vi "OUTPUT2sql.vi"() -> ()   [LabVIEW 2015]
uses:
  Controls/STORE_INPUT_NO_CLUSTER.ctl
  Controls/STORE_INPUT_INFORMATION_Cluster.ctl
  <vilib>/addons/database/Connection.llb/DB Tools Open Connec (String).vi
  <vilib>/addons/database/Connection.llb/Conn Execute.vi
  <vilib>/addons/database/Recordset.llb/Rec Destroy - Connection.vi
  <vilib>/addons/database/_DB Variant To Data/Database Variant To Data.xnode
  <vilib>/addons/database/NI_Database_API.lvlib
panel:
  out "Numeric 2":i32
  in  "stop":bool
  out "error out 5":errorcluster
  out "Numeric":i32
  out "error out 4":errorcluster
  out "error out 3":errorcluster
  out "error out 2":errorcluster
  out "error out":errorcluster
  out "Find Array":i32[](array[numeric])
  out "Input No.":string
  out "Table 2":string[][](table)
  out "ECODE":string
  in  "Input Date":timestamp format="%<%d/%m/%Y>T"
  in  "Browse":path=path "\\\\192.168.1.45\\Du Lieu Kho/Data/OutLine" caption="Path"
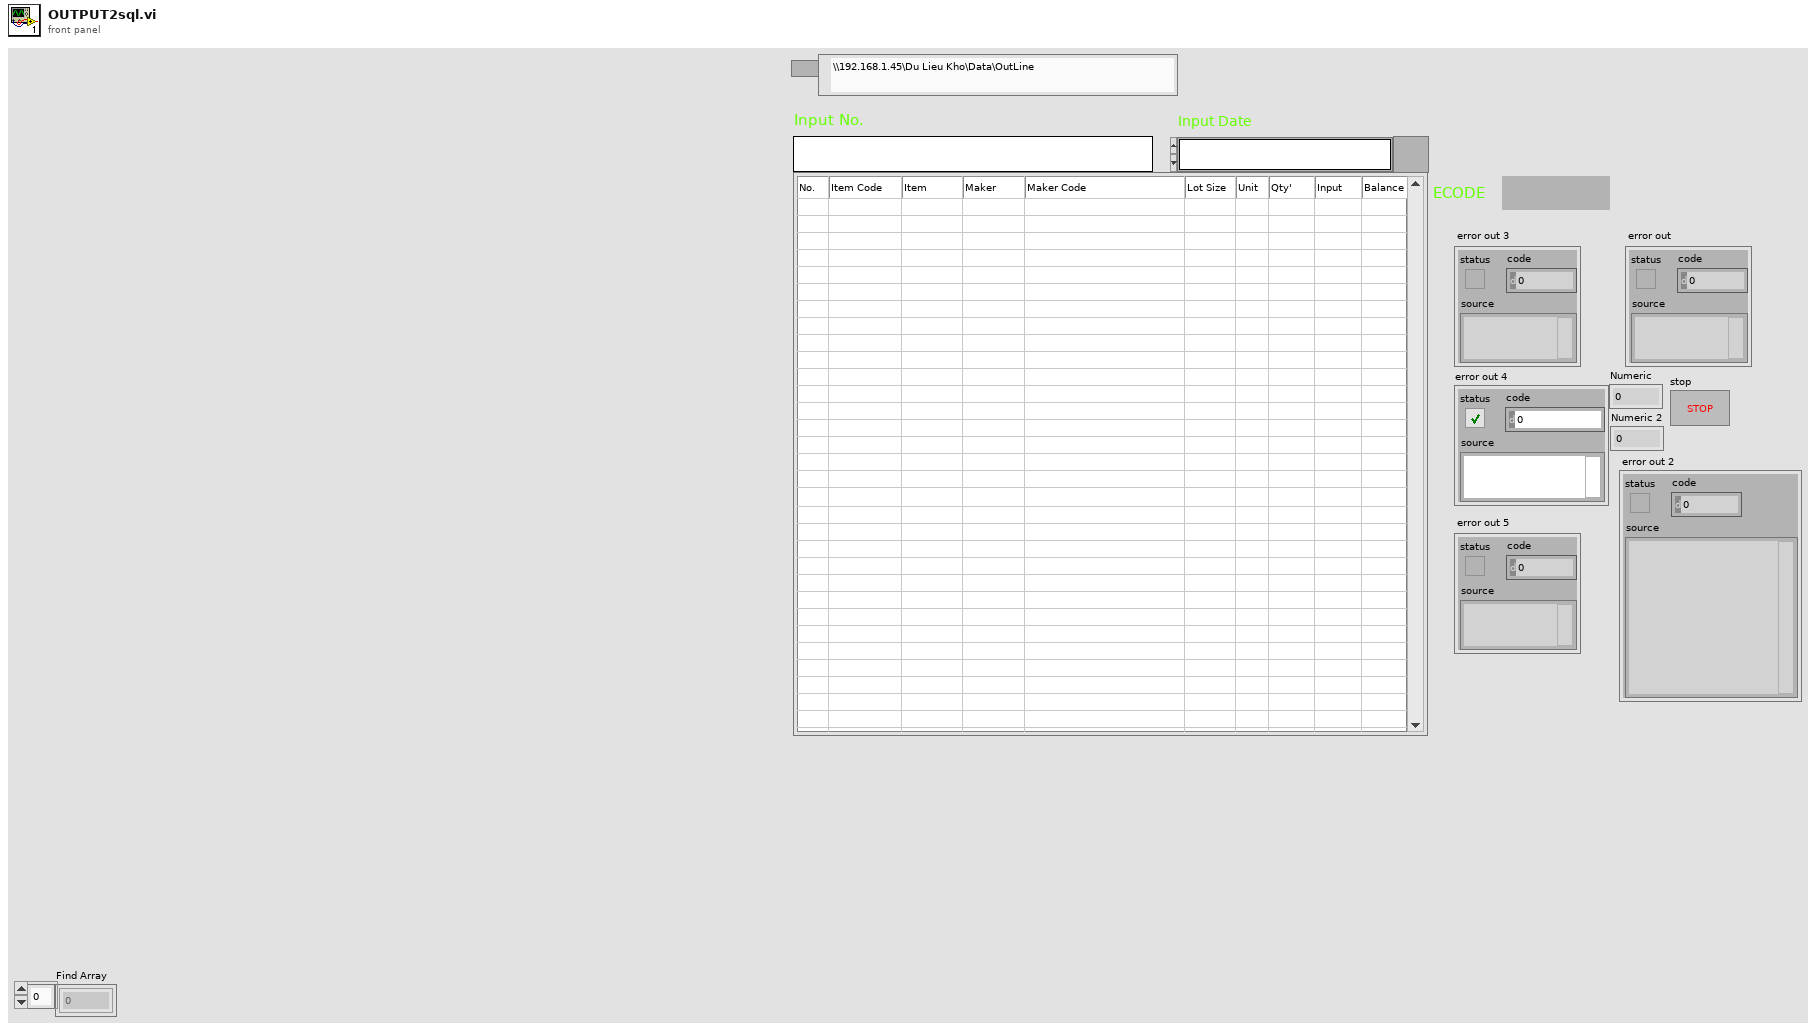
[diagram p1: front panel]
types:
  T1 = typedef "STORE_INPUT_NO_CLUSTER.ctl" = cluster{"NO":dbl, "ITEM_CODE":string, "ITEM":string, "MAKER":string, "MAKER_CODE":string, "LOT_SIZE":dbl, "UNIT":string, "QUANTITY":dbl, "INPUT":dbl, "BALANCE":dbl, "DESTINATION":string, "INVOICE_NO":string}
  T2 = enum16{"open", "replace", "create", "open or create", "replace or create", "replace or create with confirmation"}
  T3 = typedef "STORE_INPUT_INFORMATION_Cluster.ctl" = cluster{"INPUT_NO":string, "INPUT_DATE":timestamp, "ECODE":string}
  T4 = typedef "NI_Database_API.lvlib/Conn ObjectReference.ctl" = refnum<k1>
  T5 = typedef "NI_Database_API.lvlib/Rec ObjectReference.ctl" = refnum<k1>
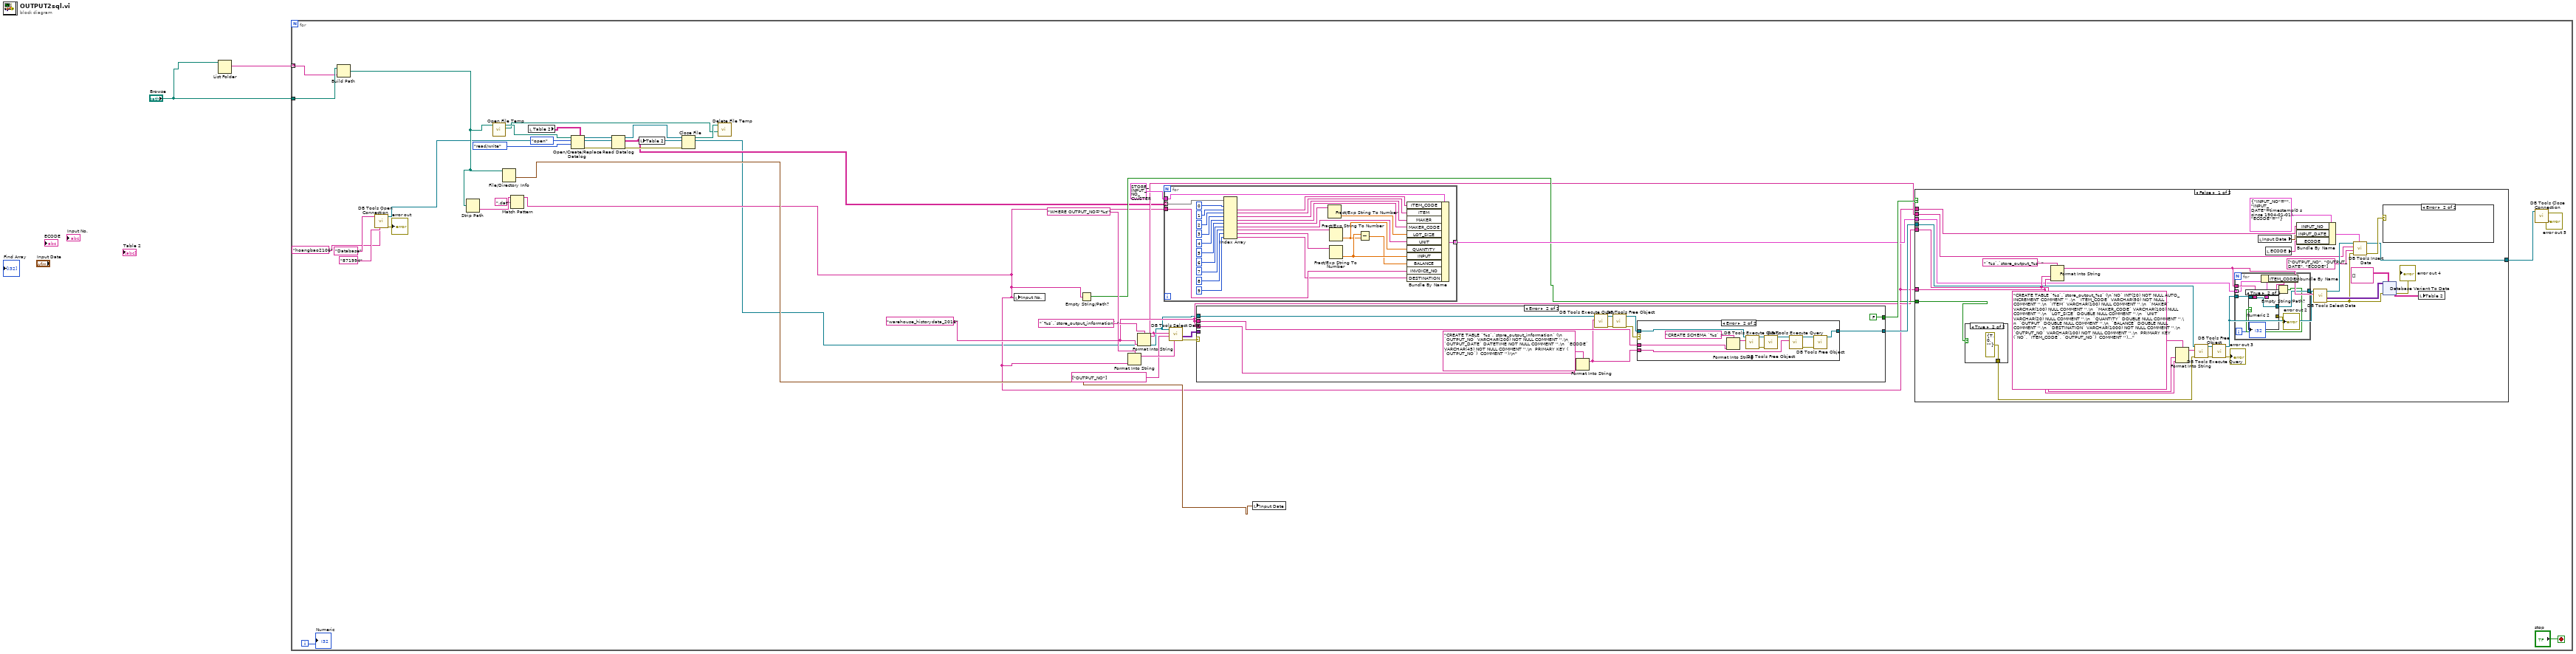
[diagram p0: block diagram]
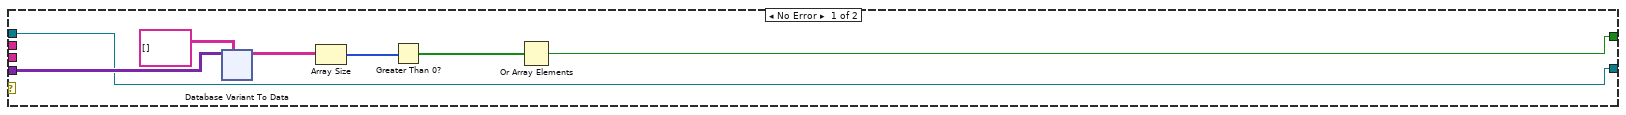
[diagram p2: hidden frame]
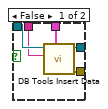
[diagram p6: hidden frame]
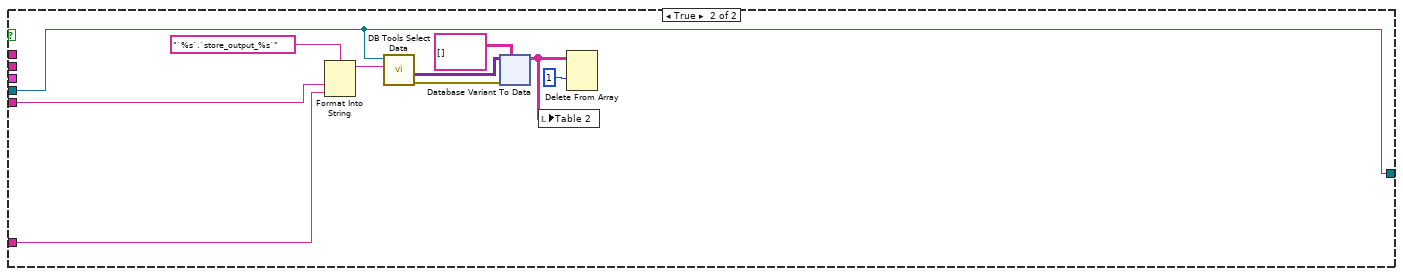
[diagram p7: hidden frame]
diagram:
  n1 = List Folder(path="Browse") -> (filenames=w2:string[])  [unwired: 3 in, 3 out]
  n2 = for {
    tunnel: "Browse" -> [w14]
    tunnel: w2 -> [w13] mode=indexing
    i -> [w11]
    stop <- "stop" stop-if-true
    w21 = "warehouse_historydata_2016"
    n3 = Build Path(base path=w14, name or relative path=w13) -> (appended path=w12:path)
    n4 = call-poly <vilib>:"DB Tools Open Connection.vi"("password"="871994" ("userID"), "userID"="hoangbao2106", "connection information"="Database" ("userID")) -> ("error out"=→"error out":errorcluster, "connection reference"=w6:T4)  [unwired: 5 in]
    n5 = Strip Path(path=w12) -> (name=w18:string)  [unwired: 1 out]
    n6 = call "Open File Temp.vi"("Path file"=w12) -> ("Source Path"=w33:path, "Temp path"=w35:path)  [unwired: 7 in, 2 out]
    n7 = File/Directory Info(path=w12) -> (last mod=w19:timestamp)  [unwired: 1 in, 6 out]
    n8 = Match Pattern(string=w18, regular expression=".dat") -> (before substring=w15:string)  [unwired: 1 in, 3 out]
    n9 = local read "Table 2"() -> (w42:string[][])
    n10 = Open/Create/Replace Datalog(5:w42, 9:enum16{"read/write", "read-only", "write-only"}."read/write" ("access (0:read/write)"), 10:T2."open" ("operation (0:open)"), 11:w35) -> (0:w37:errorcluster, 3:w39:refnum<k1>)  [unwired: 2 in, 1 out]
    n11 = Read Datalog(4:w37, 7:w39) -> (0:w36:errorcluster, 2:w16:string[][], 3:w38:refnum<k1>)  [unwired: 1 in]
    n12 = local write "Table 2"(w16) -> ()
    n13 = Close File(refnum=w38, error in=w36) -> (path=w34:path)  [unwired: 1 out]
    n14 = call "Delete File Temp.vi"("Source Path"=w33, "Temp path"=w34) -> ()  [unwired: 8 in, 2 out]
    n15 = local write "Input No."(w15) -> ()
    n16 = Empty String/Path?(string/path=w15) -> (empty?=w23:bool)
    n17 = Format Into String(format string="WHERE OUTPUT_NO='%s'", w15) -> (resulting string=w31:string)  [unwired: 2 in, 1 out]
    n18 = Format Into String(format string="`%s`.`store_output_information` ", w21) -> (resulting string=w20:string)  [unwired: 2 in, 1 out]
    n19 = for {
      tunnel: w16 -> [w68] mode=indexing
      tunnel: T1 {"NO"=0.0, "ITEM_CODE"="", "ITEM"="", "MAKER"="", "MAKER_CODE"="", "LOT_SIZE"=0.0, "UNIT"="", "QUANTITY"=0.0, "INPUT"=0.0, "BALANCE"=0.0, "DESTINATION"="", "INVOICE_NO"=""} -> [w69]
      tunnel: [w48] -> w24 mode=indexing
      tunnel: w15 -> [w47]
      n20 = Index Array(array=w68, index #1=0 ("index"), index #2=1 ("index"), index #3=2 ("index"), index #4=3 ("index"), index #5=4 ("index"), index #6=5 ("index"), index #7=6 ("index"), index #8=7 ("index"), index #9=8 ("index"), index #10=9 ("index")) -> (element #2=w57:string, element #3=w56:string, element #4=w55:string, element #5=w54:string, element #6=w53:string, element #7=w51:string, element #8=w50:string, element #9=w49:string, element #10=w43:string)  [unwired: 1 out]
      n21 = Fract/Exp String To Number(string=w53) -> (number=w52:dbl)  [unwired: 3 in, 1 out]
      n22 = Fract/Exp String To Number(string=w50) -> (number=w45:dbl)  [unwired: 3 in, 1 out]
      n23 = Fract/Exp String To Number(string=w49) -> (number=w46:dbl)  [unwired: 3 in, 1 out]
      n24 = Subtract(x=w46, y=w45) -> (x-y=w44:dbl)
      n25 = Bundle By Name(cluster=w69, "ITEM_CODE"=w57, "ITEM"=w56, "MAKER"=w55, "MAKER_CODE"=w54, "LOT_SIZE"=w52, "UNIT"=w51, "QUANTITY"=w45, "INPUT"=w46, "BALANCE"=w44, "INVOICE_NO"=w47, "DESTINATION"=w43) -> (w48:T1)
    }
    n26 = call <vilib>:"DB Tools Select Data.vi"("condition"=w31, "columns"=string[] ["OUTPUT_NO"], "table"=w20, "connection reference"=w6) -> ("error out"=w27:errorcluster, "data"=w30:variant[][])  [unwired: 2 in, 1 out]
    n27 = case shown="Error" w27 {
      tunnel: w30 -> [w76 _]
      tunnel: [w71 FALSE] -> w28
      tunnel: w6 -> [w70 w128]
      tunnel: [w70 w124] -> w26
      tunnel: w21 -> [_ w126]
      tunnel: w21 -> [_ w122]
      frame No Error {
        n28 = xnode "Database Variant To Data"("database variant"=w76, "type"=string[][] []) -> ("data"=w74:string[][])  [unwired: 1 in, 1 out]
        n29 = Array Size(array=w74) -> (size(s)=w73:i32[])
        n30 = Greater Than 0?(x=w73) -> (x > 0?=w72:bool[])
        n31 = Or Array Elements(Boolean array=w72) -> (logical OR=w71:bool)
      }
      frame Error {
        n32 = Format Into String(format string="CREATE TABLE `%s`.`store_output_information` (\n  `OUTPUT_NO` VARCHAR(200) NOT NULL COMMENT '',\n  `OUTPUT_DATE` DATETIME NOT NULL COMMENT '',\n  `ECODE` VARCHAR(45) NOT NULL COMMENT '',\n  PRIMARY KEY (  `OUTPUT_NO`)  COMMENT '');\n", w122) -> (resulting string=w121:string)  [unwired: 2 in, 1 out]
        n33 = call-poly <vilib>:"DB Tools Execute Query.vi"("SQL query"=w121, "connection reference"=w128) -> ("error out"=w130:errorcluster, "recordset reference"=w131:T5)  [unwired: 6 in]
        n34 = call-poly <vilib>:"DB Tools Free Object.vi"("error in (no error)"=w130, "recordset reference"=w131) -> ("error out"=w127:errorcluster, "connection reference"=w125:T4)  [unwired: 8 in]
        n35 = case shown="Error" w127 {
          tunnel: w125 -> [w132 w143]
          tunnel: w126 -> [_ w141]
          tunnel: w121 -> [_ w135]
          tunnel: [w132 w134] -> w124
          frame No Error {
          }
          frame Error {
            n36 = Format Into String(format string="CREATE SCHEMA `%s` ;" ("SQL query"), w141) -> (resulting string=w133:string)  [unwired: 2 in, 1 out]
            n37 = call-poly <vilib>:"DB Tools Execute Query.vi"("SQL query"=w133, "connection reference"=w143) -> ("error out"=w139:errorcluster, "recordset reference"=w140:T5)  [unwired: 6 in]
            n38 = call-poly <vilib>:"DB Tools Free Object.vi"("error in (no error)"=w139, "recordset reference"=w140) -> ("connection reference"=w136:T4)  [unwired: 8 in, 1 out]
            n39 = call-poly <vilib>:"DB Tools Execute Query.vi"("SQL query"=w135, "connection reference"=w136) -> ("error out"=w138:errorcluster, "recordset reference"=w137:T5)  [unwired: 6 in]
            n40 = call-poly <vilib>:"DB Tools Free Object.vi"("error in (no error)"=w138, "recordset reference"=w137) -> ("connection reference"=w134:T4)  [unwired: 8 in, 1 out]
          }
        }
      }
    }
    n41 = local write "Input Date"(w19) -> ()
    n42 = case shown="False" w28 {
      tunnel: w26 -> [w172 w241]
      tunnel: w21 -> [w167 w235]
      tunnel: w15 -> [w166 w236]
      tunnel: [w155 w241] -> w5
      tunnel: w24 -> [w165 _]
      tunnel: w20 -> [w158 _]
      tunnel: w15 -> [w154 _]
      tunnel: w23 -> [w148 _]
      frame False {
        n43 = case shown="True" w148 {
          tunnel: [_ errorcluster {"status"=TRUE, "code"=0, "source"=""} ("error constant")] -> w147
          frame False {
          }
          frame True {
          }
        }
        n44 = Format Into String(format string="`%s`.`store_output_%s` " ("SQL query"), w167, w166) -> (resulting string=w161:string)  [unwired: 2 in, 1 out]
        n45 = Format Into String(format string="CREATE TABLE `%s`.`store_output_%s` (\n`NO` INT(20) NOT NULL AUTO_INCREMENT COMMENT '' ,\n  `ITEM_CODE` VARCHAR(50) NOT NULL COMMENT '',\n  `ITEM` VARCHAR(100) NULL COMMENT '',\n  `MAKER` VARCHAR(100) NULL COMMENT '',\n  `MAKER_CODE` VARCHAR(100) NULL COMMENT '',\n  `LOT_SIZE` DOUBLE NULL COMMENT '',\n  `UNIT` VARCHAR(20) NULL COMMENT '',\n  `QUANTITY` DOUBLE NULL COMMENT '',\n  `OUTPUT` DOUBLE NULL COMMENT '',\n  `BALANCE` DOUBLE NULL COMMENT '',\n  `DESTINATION` VARCHAR(1000) NOT NULL COMMENT '',\n  `OUTPUT_NO` VARCHAR(100) NOT NULL COMMENT '',\n  PRIMARY KEY (`NO`, `ITEM_CODE`, `OUTPUT_NO`)  COMMENT '');\n" ("SQL query"), w167, w166) -> (resulting string=w160:string)  [unwired: 2 in, 1 out]
        n46 = call-poly <vilib>:"DB Tools Execute Query.vi"("error in (no error)"=w147, "SQL query"=w160, "connection reference"=w172) -> ("error out"=w169:errorcluster, "recordset reference"=w170:T5)  [unwired: 5 in]
        n47 = call-poly <vilib>:"DB Tools Free Object.vi"("error in (no error)"=w169, "recordset reference"=w170) -> ("error out"=→"error out 3":errorcluster, "connection reference"=w146:T4)  [unwired: 8 in]
        n48 = for {
          tunnel: w146 -> [w225]
          tunnel: w161 -> [w224]
          tunnel: w165 -> [w221] mode=indexing
          tunnel: [w223] -> _
          i -> [w218]
          n49 = Unbundle By Name(w221) -> ("ITEM_CODE"=w220:string)
          n50 = Empty String/Path?(string/path=w220) -> (empty?=w219:bool)
          n51 = case shown="True" w219 {
            tunnel: w225 -> [w230 w231]
            tunnel: w224 -> [w229 _]
            tunnel: [w228 w231] -> w223
            tunnel: [w227 _] -> w222
            tunnel: w221 -> [w226 _]
            frame False {
              n52 = call <vilib>:"DB Tools Insert Data.vi"("data"=w226, "table"=w229, "connection reference"=w230) -> ("error out"=w227:errorcluster, "connection reference out"=w228:T4)  [unwired: 7 in]
            }
            frame True {
            }
          }
          "error out 2" <- w222
          "Numeric 2" <- w218
        }
        n53 = local read "Input Date"() -> (w153:timestamp)
        n54 = local read "ECODE"() -> (w152:string)
        n55 = Bundle By Name(cluster=T3 {"INPUT_NO"="", "INPUT_DATE"=timestamp(0 s since 1904-01-01), "ECODE"=""} ("INVOICE_INFORMATION_Cluster"), "INPUT_NO"=w154, "INPUT_DATE"=w153, "ECODE"=w152) -> (w151:T3)
        n56 = call <vilib>:"DB Tools Select Data.vi"("table"=w161, "connection reference"=w146) -> ("error out"=w157:errorcluster, "data"=w164:variant[][], "connection reference out"=w159:T4)  [unwired: 4 in]
        n57 = call <vilib>:"DB Tools Insert Data.vi"("data"=w151, "error in (no error)"=w157, "columns"=string[] ["OUTPUT_NO", "OUTPUT_DATE", "ECODE"], "table"=w158, "connection reference"=w159) -> ("error out"=w156:errorcluster, "connection reference out"=w155:T4)  [unwired: 5 in]
        n58 = case shown="Error" w156 {
          frame No Error {
          }
          frame Error {
          }
        }
        n59 = xnode "Database Variant To Data"("database variant"=w164, "error in (no error)"=w157, "type"=string[][] []) -> ("data"=w162:string[][], "error out"=→"error out 4":errorcluster)
        n60 = local write "Table 2"(w162) -> ()
      }
      frame True {
        n61 = Format Into String(format string="`%s`.`store_output_%s`", w235, w236) -> (resulting string=w234:string)  [unwired: 2 in, 1 out]
        n62 = call <vilib>:"DB Tools Select Data.vi"("table"=w234, "connection reference"=w241) -> ("error out"=w238:errorcluster, "data"=w240:variant[][])  [unwired: 4 in, 1 out]
        n63 = xnode "Database Variant To Data"("database variant"=w240, "error in (no error)"=w238, "type"=string[][] []) -> ("data"=w233:string[][])  [unwired: 1 out]
        n64 = local write "Table 2"(w233) -> ()
        n65 = Delete From Array(array=w233, index (row)=1) -> ()  [unwired: 2 in, 2 out]
      }
    }
    n66 = call <vilib>:"DB Tools Close Connection.vi"("connection reference"=w5) -> ("error out"=→"error out 5":errorcluster)  [unwired: 6 in]
    "Numeric" <- w11
  }
